vi "StopServer.vi"(8 "error in (no error)":errorcluster, 11 "Server Id":T1) -> (0 "error out":errorcluster)   [LabVIEW 2019, in "gprc-support.lvlib"]
uses:
  gprc-support.lvlib
  grpcId.ctl
  home/lvuser/liblabview_grpc_server.so
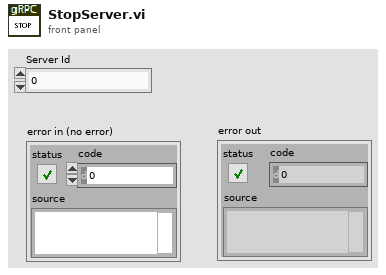
[diagram p1: front panel]
types:
  T1 = typedef "gprc-support.lvlib/grpcId.ctl" = u64
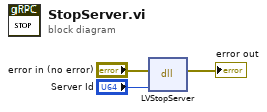
[diagram p0: block diagram]
diagram:
  n1 = dll-call lib="home/lvuser/liblabview_grpc_server.so" fn="LVStopServer"(error in="error in (no error)", "server"="Server Id") -> (error out=→"error out":errorcluster)  [unwired: 4 in, 1 out]
